vi "getTestList.vi"(8 "error in (no error)":errorcluster, 10 "listaPruebas":refnum<vi>, 11 "Sonometro in":refnum<class "Sonometro.lvclass">) -> (0 "error out":errorcluster, 2 "listaDePruebas":refnum<class "Prueba.lvclass">[](array[class]), 3 "Sonometro out":refnum<class "Sonometro.lvclass">)   [LabVIEW 2019, in "Sonometro.lvclass"]
uses:
  Sonometro.lvclass
  Pruebas/Prueba/Prueba.lvclass
  Sonometro.lvclass/Sonometro.ctl
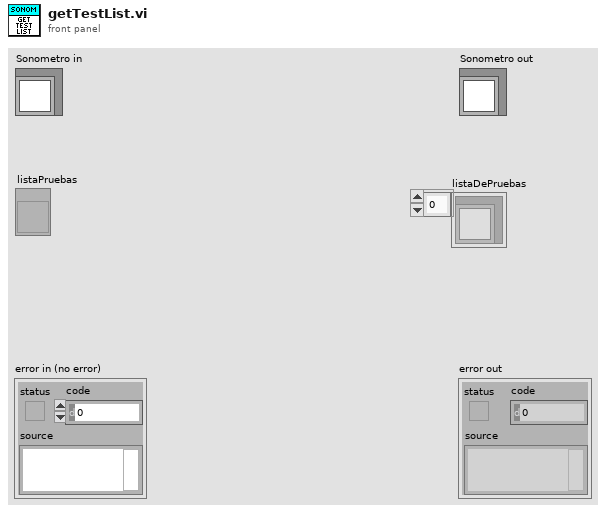
[diagram p1: front panel]
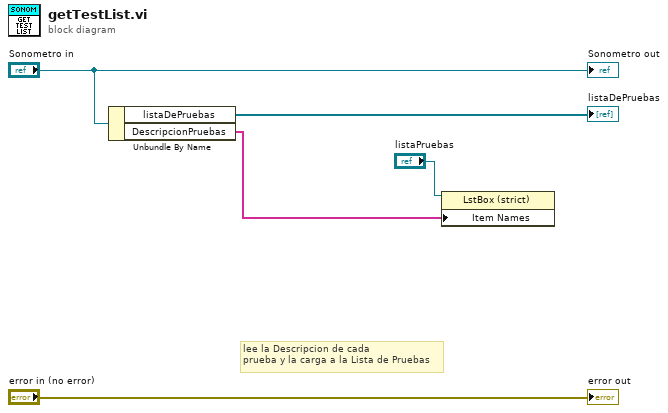
[diagram p0: block diagram]
diagram:
  # "lee la Descripcion de cada\nprueba y la carga a la Lista de Pruebas"
  n1 = Unbundle By Name("Sonometro in") -> ("listaDePruebas"=→"listaDePruebas":refnum<class "Prueba.lvclass">[], "DescripcionPruebas"=w1:string[])
  n2 = property class="LstBox (strict)"(reference="listaPruebas", "Item Names"=w1) -> ()  [unwired: 1 in, 2 out]
  "error out" <- "error in (no error)"
  "Sonometro out" <- "Sonometro in"
